vi "StopSignal-Create.vi"(8 "error in (no error)":errorcluster) -> (0 "error out":errorcluster, 3 "StopSignal":T1)   [LabVIEW 2017, in "StopSignal.lvlib"]
uses:
  StopSignal.lvlib
  Typedef/Def-StopSignalData.ctl
  Typedef/StopSignal.ctl
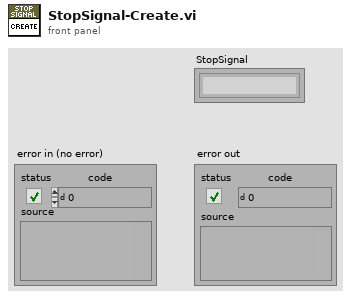
[diagram p1: front panel]
types:
  T1 = typedef "StopSignal.lvlib/StopSignal.ctl" = refnum<k1>
  T2 = typedef "StopSignal.lvlib/Def-StopSignalData.ctl" = cluster{"StopEvent":refnum<user-event>, "StopNotifier":refnum<notifier>}
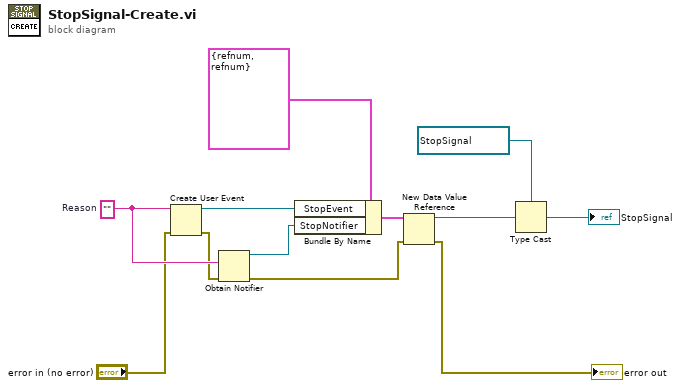
[diagram p0: block diagram]
diagram:
  w6 = T1 refnum items=["StopSignal"] ("StopSignal")
  w8 = ""  # Reason
  n1 = Create User Event(user event datatype=w8, error in="error in (no error)") -> (user event=w11:refnum<user-event>, error out=w2:errorcluster)
  n2 = Obtain Notifier(notification data type=w8, error in (no error)=w2) -> (notifier out=w10:refnum<notifier>, error out=w3:errorcluster)  [unwired: 2 in, 1 out]
  n3 = Bundle By Name(cluster=T2 {"StopEvent"=refnum, "StopNotifier"=refnum} ("Def-xxxxx"), "StopEvent"=w11, "StopNotifier"=w10) -> (w9:T2)
  n4 = New Data Value Reference(data value=w9, error in=w3) -> (data value reference=w7:refnum<data-value>, error out=→"error out":errorcluster)
  n5 = Type Cast(type=w6, x=w7) -> (*(type *) &x=→"StopSignal":T1)
